vi "Applied Scale and Offset to Signal.vi"(9 "Scale":dbl[](array[numeric]), 10 "Offset":dbl[](array[numeric]), 11 "Raw Data":waveform(dbl)[](array[waveform])) -> (3 "Conditioned Signal":waveform(dbl)[](array[waveform]))   [LabVIEW 2021]
doc: "Apply scale and offset to raw data"
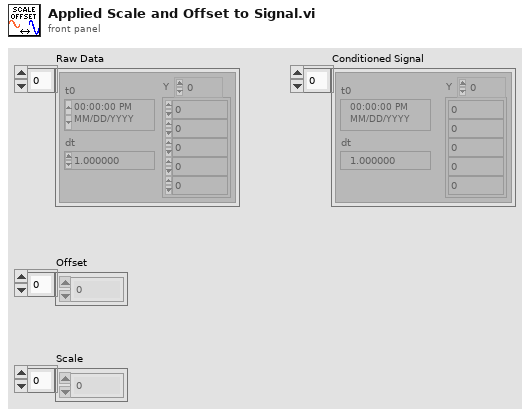
[diagram p1: front panel]
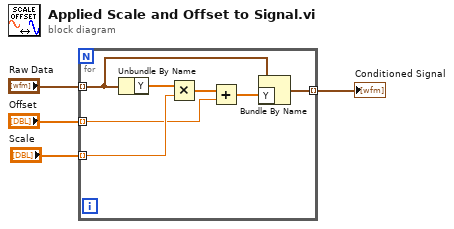
[diagram p0: block diagram]
diagram:
  n1 = for {
    tunnel: "Raw Data" -> [w10] mode=indexing
    tunnel: "Offset" -> [w6] mode=indexing
    tunnel: [w11] -> w1 mode=indexing
    tunnel: "Scale" -> [w9] mode=indexing
    n2 = Unbundle By Name(w10) -> ("Y"=w8:dbl[])
    n3 = Multiply(x=w8, y=w9) -> (x*y=w7:dbl[])
    n4 = Add(x=w7, y=w6) -> (x+y=w5:dbl[])
    n5 = Bundle By Name(cluster=w10, "Y"=w5) -> (w11:waveform(dbl))
  }
  "Conditioned Signal" <- w1
